vi "Server Thread Handle Message.vi"(2 "error in":errorcluster, 3 "Server Thread":cluster{"connection ID":refnum<k5>}, 4 "Timestamp":dbl format="%#_13g", 5 "Vision Message":cluster{"Type":string, "Message":string}) -> (0 "error out":errorcluster, 1 "Targets":cluster{"X":dbl, "Y":dbl, "Z":dbl}[](array[cluster]))   [LabVIEW 2016]
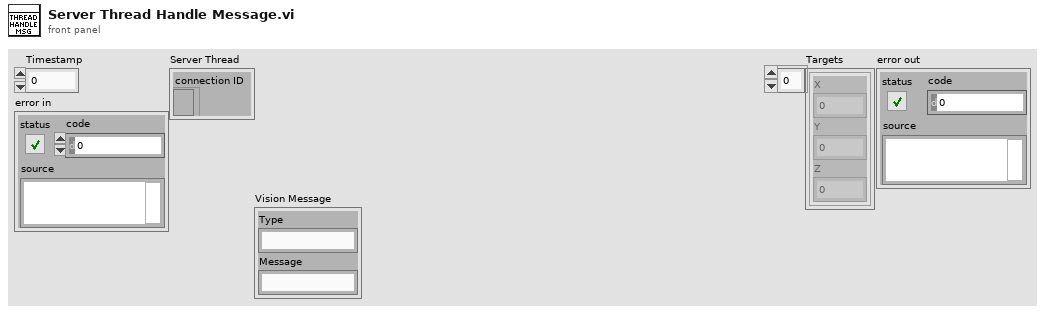
[diagram p1: front panel]
types:
  T1 = cluster{"CapturedAgoMs":i32, "Valid?":bool, "CapturedAtTimestamp":dbl, "Targets":cluster{"X":dbl, "Y":dbl, "Z":dbl}[]}
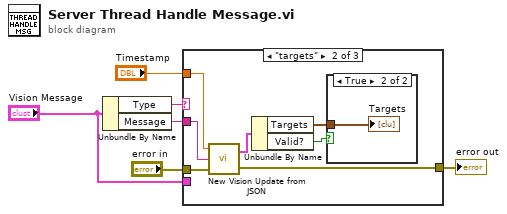
[diagram p0: block diagram]
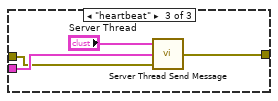
[diagram p4: hidden frame]
diagram:
  n1 = Unbundle By Name("Vision Message") -> ("Type"=w6:string, "Message"=w5:string)
  n2 = case shown="\"targets\"" w6 {
    tunnel: w5 -> [_ w13 _]
    tunnel: "Timestamp" -> [_ w14 _]
    tunnel: "error in" -> [w7 w12 w17]
    tunnel: "Vision Message" -> [_ _ w18]
    tunnel: [w7 w8 w16] -> w1
    frame Default {
    }
    frame "targets" {
      n3 = call "New Vision Update from JSON.vi"("error in"=w12, "JSON string"=w13, "Current Time (ms)"=w14) -> ("error out"=w8:errorcluster, "Vision Update"=w11:T1)
      n4 = Unbundle By Name(w11) -> ("Targets"=w9:cluster{"X":dbl, "Y":dbl, "Z":dbl}[], "Valid?"=w10:bool)
      n5 = case shown="True" w10 {
        tunnel: w9 -> [_ w15]
        frame False {
        }
        frame True {
          "Targets" <- w15
        }
      }
    }
    frame "heartbeat" {
      n6 = call "Server Thread Send Message.vi"("error in"=w17, "Vision Message"=w18, "Server Thread"="Server Thread") -> ("error out"=w16:errorcluster)
    }
  }
  "error out" <- w1
